vi "SLL DE AI Continuous Engine.vi"(8 "error in (no error)":errorcluster, 11 "Delay (ms)":u32=100) -> (0 "error out":errorcluster)   [LabVIEW 2013]
doc: "Copyright © 2005, Soliton Technologies.\nAll rights reserved."
uses:
  Controls/SLL DE DAQ Engine Options.ctl
  Controls/SLL DE DAQ Engine Channel Types.ctl
  Controls/SLL DE Circular Buffer Options.ctl
  Controls/SLL DE DAQ Global Options.ctl
  Controls/SLL DE DAQ Global Elements.ctl
  Controls/SLL DE DAQ Parameters LV2Global Options.ctl
  <vilib>/DAQmx/configure/timing.llb/DAQmx Timing (Sample Clock).vi
  <vilib>/DAQmx/read.llb/DAQmx Read (Analog 1D Wfm NChan NSamp).vi
  <vilib>/DAQmx/configure/trigger.llb/DAQmx Start Trigger (Digital Edge).vi
panel:
  in  "Data Cluster":T1={"Array of Tasks"=[], "Channel Order"=[], "AI Data"=[], "# Samples"=0, "# Channels"=0, "Time Increments"=[], "AI Cont. Parameters"={"AI Sampling Rate"=1000.0, "MvgAVG Window Size"=1000, "Enable Filter"=TRUE, "Enable MvgAVG"=TRUE}}
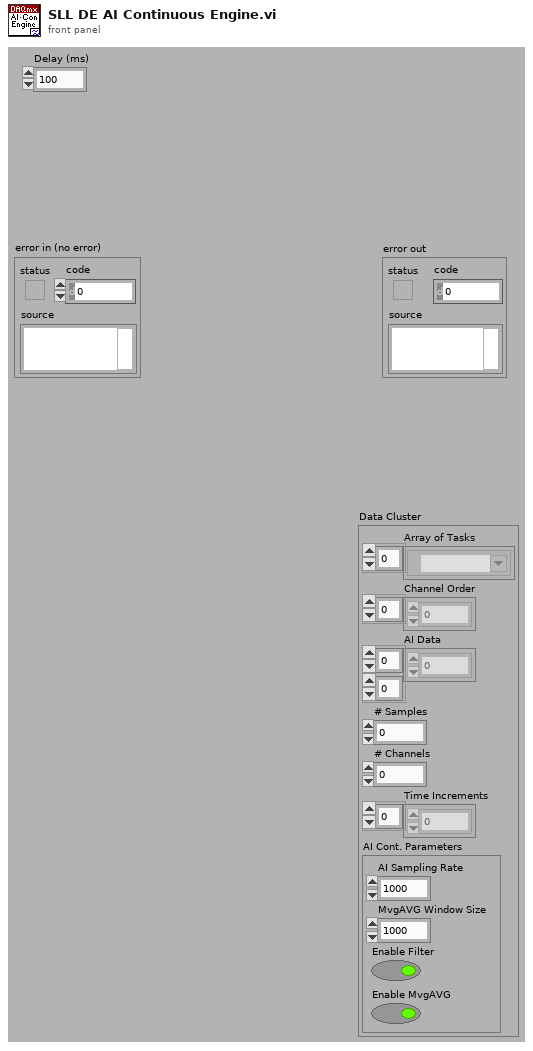
[diagram p1: front panel]
types:
  T1 = cluster{"Array of Tasks":refnum<k21>[], "Channel Order":i32[], "AI Data":dbl[][], "# Samples":i32, "# Channels":i32, "Time Increments":dbl[], "AI Cont. Parameters":cluster{"AI Sampling Rate":dbl, "MvgAVG Window Size":i32, "Enable Filter":bool, "Enable MvgAVG":bool}}
  T2 = typedef "SLL DE DAQ Engine Options.ctl" = enum16{">Init", ">Safe Mode", ">Poll", ">Error", ">Exit", ">Restart", ">DI", ">DO", ">AI", ">AO", ">Start Task", ">Stop Task"}
  T3 = typedef "SLL DE DAQ Parameters LV2Global Options.ctl" = enum16{"Read", "Write"}
  T4 = typedef "SLL DE DAQ Global Options.ctl" = enum16{"Init", "Write 1", "Read 1", "Write Array", "Read Array", "Clear"}
  T5 = typedef "SLL DE Circular Buffer Options.ctl" = enum16{"Initialize", "Init Pointer X", "Write", "Read Single Value", "Read Pointer X (Multi Value)", "Clear Data"}
  T6 = typedef "SLL DE DAQ Engine Channel Types.ctl" = enum16{"Analog Input", "Analog Output", "Digital Input", "Digital Output"}
  T7 = typedef "SLL DE DAQ Global Elements.ctl" = enum16{"AI Error", "AO Error", "DI Error", "DO Error", "AI Restart", "DI Restart", "AI Running", "AO Running", "DI Running", "DO Running", "DAQ Exit?"}
  T8 = typedef "SLL DE DAQ Engine Parameters.ctl" = cluster{"Enable Engines":cluster{"AI Enable":bool, "AO Enable":bool, "DI Enable":bool, "DO Enable":bool}, "DAQ Control Type":cluster{"Analog Input":enum16{"Finite", "Continuous", "Driver"}, "Analog Output":enum16{"Finite", "Continuous", "Driver"}, "Digital Input":enum16{"Finite", "Continuous", "Driver"}, "Digital Output":enum16{"Finite", "Continuous", "Driver"}}, "DAQ Parameters":cluster{"AI Sampling Rate (Samples/Sec)":dbl, "MvgAVG Window Size (# of Points)":i32, "Enable Filter":bool, "Enable MvgAVG":bool, "Circular Buffer Size (Sec)":dbl, "AO Sampling Rate (Samples/Sec)":dbl, "Graph Update Rate (Samples/Sec)":dbl, "File Logging Rate (Samples/Sec)":i32}, "AO Safe Values":cluster{"Analog Outputs Name":T9, "Analog Outputs Safe Value":dbl}[], "DO Safe Values":cluster{"Digital Outputs Name":T10, "Digital Outputs Safe Value":bool}[], "DO Interconnected Lines":cluster{"First DO Line":string, "Second DO Line":string}[], "AI Channels Unit":cluster{"Channel Name":T11, "Channel Type":T12}[], "Units Information":cluster{"Channel Type":T12, "Unit Text":string, "Maximum":dbl, "Minmum":dbl, "Increments":dbl}[]}
  T9 = typedef "SLL DE List of Analog Outputs.ctl" = enum16{"None"}
  T10 = typedef "SLL DE List of Digital Outputs.ctl" = enum16{"STATION1_START TEST", "STATION1_STOP TEST", "STATION1_LIGHT1", "STATION1_LIGHT2", "STATION1_LIGHT3", "STATION1_SELECT_TEST", "STATION2_START TEST", "STATION2_STOP TEST", "STATION2_LIGHT1", "STATION2_LIGHT2", "STATION2_LIGHT3", "STATION2_SELECT_TEST", "STATION3_START TEST", "STATION3_STOP TEST", "STATION3_LIGHT1", "STATION3_LIGHT2", "STATION3_LIGHT3", "STATION3_SELECT_TEST", "STATION4_START TEST", "STATION4_STOP TEST", "STATION4_LIGHT1", "STATION4_LIGHT2", "STATION4_LIGHT3", "STATION4_SELECT_TEST"}
  T11 = typedef "SLL DE List of Analog Inputs.ctl" = enum16{"None"}
  T12 = typedef "SLL DE List of AI Channel Type.ctl" = enum16{"Pressure", "Flow", "Temperature", "Time Scale", "Voltage", "Current", "Frequency", "Sound", "Speed", "Torque", "Distance", "Channel Type 1", "Channel Type 2", "Channel Type 3"}
  T13 = enum16{"Left Button", "Center Button", "Right Button", "Window Close"}
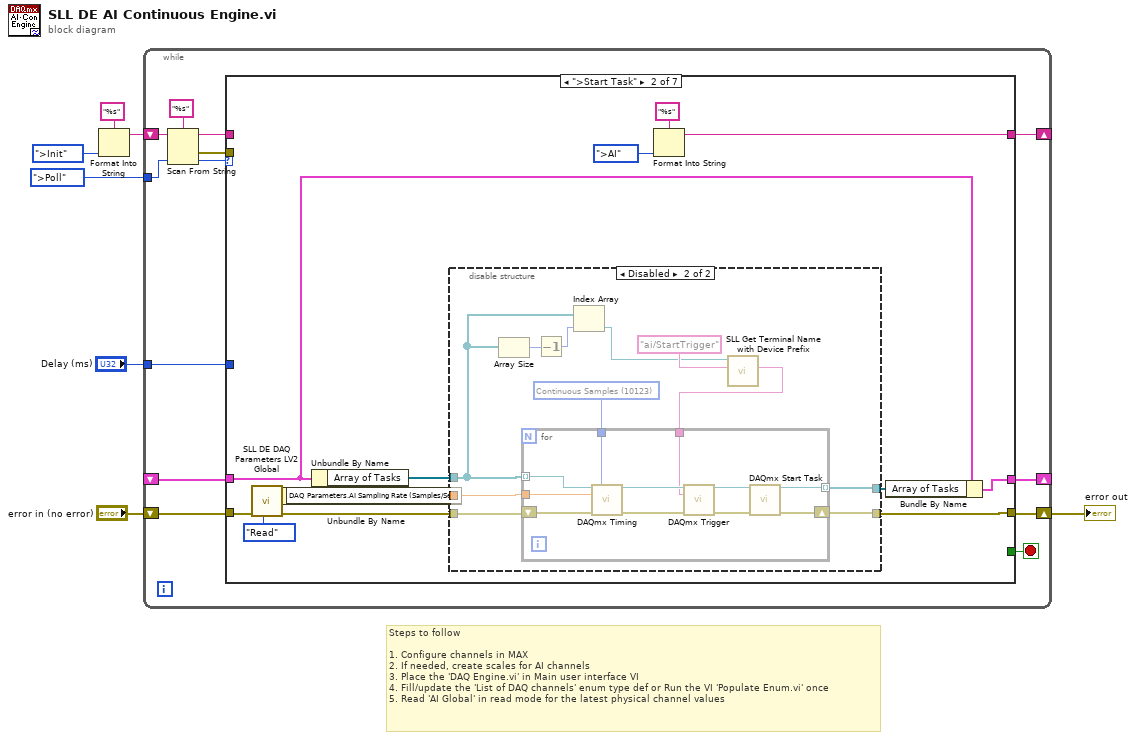
[diagram p0: block diagram]
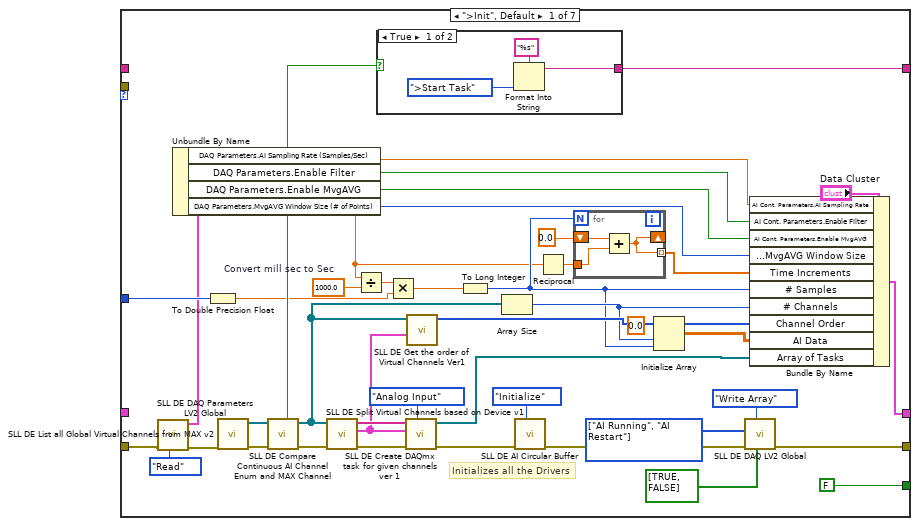
[diagram p2: hidden frame]
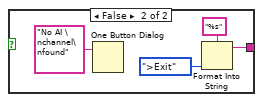
[diagram p3: hidden frame]
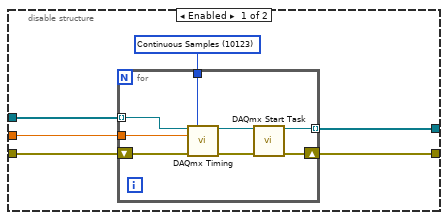
[diagram p4: hidden frame]
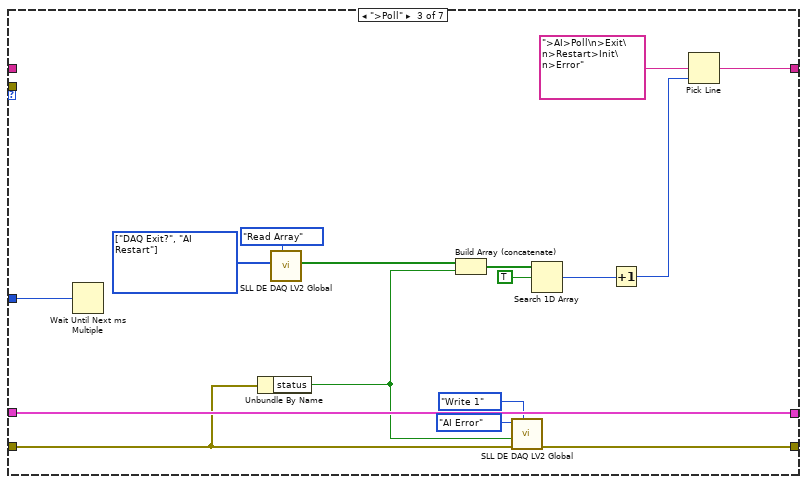
[diagram p5: hidden frame]
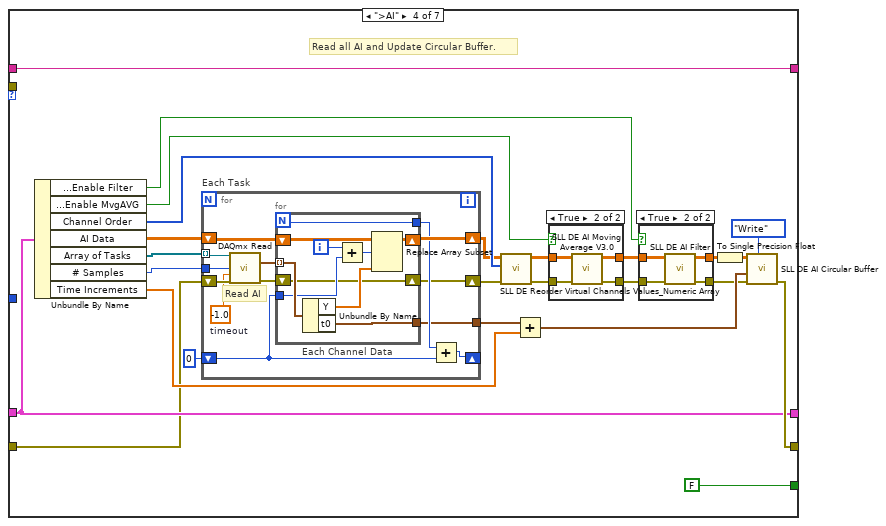
[diagram p6: hidden frame]
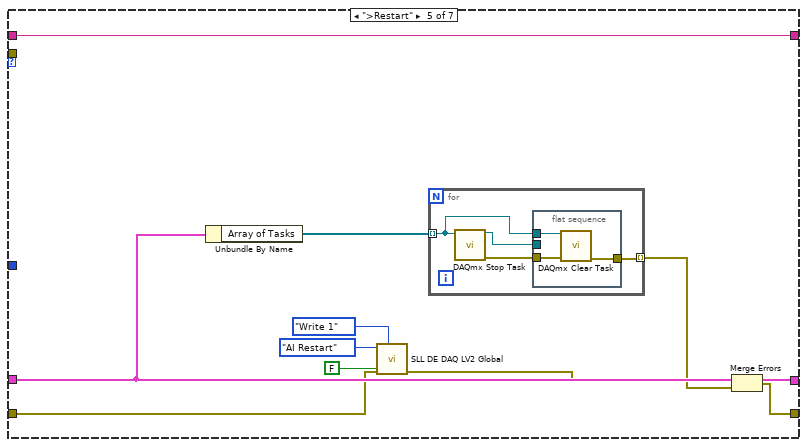
[diagram p9: hidden frame]
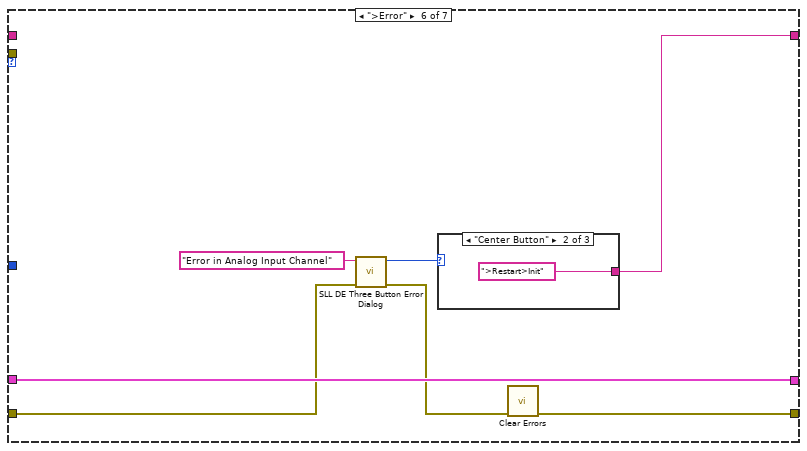
[diagram p10: hidden frame]
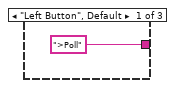
[diagram p11: hidden frame]
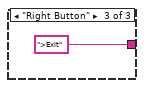
[diagram p12: hidden frame]
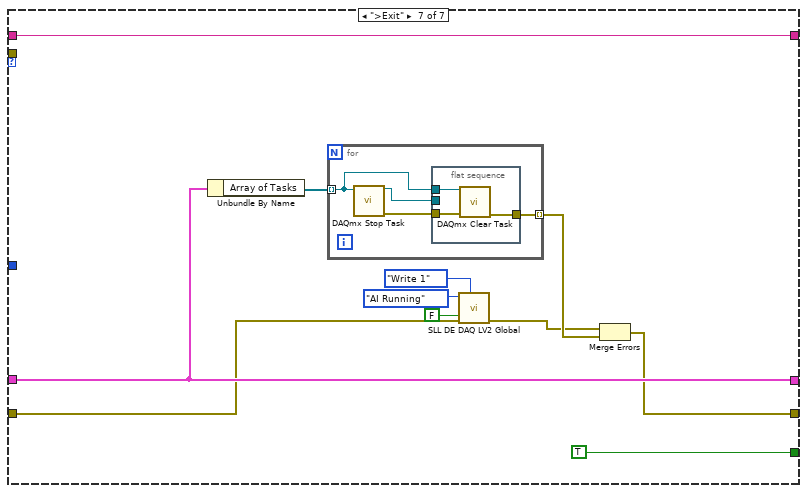
[diagram p13: hidden frame]
diagram:
  # "Steps to follow\n\n1.\tConfigure channels in MAX\n2.\tIf needed, create scales for AI channels\n3.\tPlace the 'DAQ Engine.vi' in Main user interface VI\n4.\tFill/update the 'List of DAQ channels' enum type def or Run the VI 'Populate Enum.vi' once\n5.\tRead 'AI Global' in read mode for the latest physical channel values"
  n1 = Format Into String(format string="%s", SLL_DE_DAQ_Engine_Options.">Init" ("DAQ Options")) -> (resulting string=w3:string)  [unwired: 2 in, 1 out]
  n2 = while {
    shift-right: [w19] -> w6
    shift-left: "error in (no error)" -> [w20]
    shift-right: [w18] -> _
    shift-left: _ -> [w17]
    shift-right: [w13] -> _
    shift-left: w3 -> [w16]
    tunnel: "Delay (ms)" -> [w11]
    tunnel: SLL_DE_DAQ_Engine_Options.">Poll" ("DAQ Options") -> [w9]
    stop <- w12 stop-if-true
    n3 = Scan From String(format string="%s", input string=w16, default 1=w9) -> (remaining string=w15:string, error out=w14:errorcluster, output 1=w10:T2)  [unwired: 2 in, 1 out]
    n4 = case shown="\">Start Task\"" w10 {
      tunnel: w20 -> [w24 w76 w127 w151 w201 w215 w224]
      tunnel: [w56 w81 w126 w159 w197 w217 w229] -> w19
      tunnel: [w62 w82 w137 w156 w206 w220 w232] -> w18
      tunnel: w17 -> [_ w83 w137 w156 w206 w220 w232]
      tunnel: w15 -> [_ _ _ w161 w200 _ w234]
      tunnel: w14 -> [_ _ _ _ _ _ _]
      tunnel: [w59 w78 w131 w161 w200 w216 w234] -> w13
      tunnel: [FALSE _ _ FALSE _ _ TRUE] -> w12
      tunnel: w11 -> [w40 _ w130 _ _ _ _]
      frame ">Init", Default {
        w55 = T7[] [enum."AI Running", enum."AI Restart"] items=["AI Error", "AO Error", "DI Error", "DO Error", "AI Restart", "DI Restart", "AI Running", "AO Running", "DI Running", "DO Running", "DAQ Exit?"] ("Elements Array")
        w42 = 1000.0  # Convert mill sec to Sec
        # "Initializes all the Drivers"
        n5 = call "SLL DE DAQ Parameters LV2 Global.vi"("Option"=SLL_DE_DAQ_Parameters_LV2Global_Options."Read", "Error in (no error)"=w24) -> ("Error out"=w23:errorcluster, "Global Info"=w22:T8)  [unwired: 8 in]
        n6 = Unbundle By Name(w22) -> ("DAQ Parameters.AI Sampling Rate (Samples/Sec)"=w30:dbl, "DAQ Parameters.Enable Filter"=w29:bool, "DAQ Parameters.Enable MvgAVG"=w28:bool, "DAQ Parameters.MvgAVG Window Size (# of Points)"=w27:i32)
        n7 = To Double Precision Float(number=w40) -> (double precision float=w39:dbl)
        n8 = call "SLL DE List all Global Virtual Channels from MAX v2.vi"("error in (no error)"=w23) -> ("error out"=w46:errorcluster, "Analog Input"=w44:refnum<k21>[])  [unwired: 4 in, 5 out]
        n9 = call "SLL DE Compare Continuous AI Channel Enum and MAX Channel.vi"("error in (no error)"=w46, "Analog Input Channels"=w44) -> ("error out"=w45:errorcluster, "Channels Out"=w38:refnum<k21>[], "Pass?"=w43:bool)  [unwired: 7 in]
        n10 = call "SLL DE Split Virtual Channels based on Device v1.vi"("error in (no error)"=w45, "GlobalChans"=w38) -> ("error out"=w51:errorcluster, "Channel Array"=w48:cluster{"Device Channel List":string[]}[], "Devices Names"=w52:string[])  [unwired: 7 in]
        n11 = Divide(x=w30, y=w42) -> (x/y=w41:dbl)
        n12 = case shown="True" w43 {
          tunnel: [w66 w70] -> w59
          frame True {
            n13 = Format Into String(format string="%s", SLL_DE_DAQ_Engine_Options.">Start Task" ("DAQ Options")) -> (resulting string=w66:string)  [unwired: 2 in, 1 out]
          }
          frame False {
            n14 = One Button Dialog(message="No AI \nchannel\nfound") -> ()  [unwired: 1 in, 1 out]
            n15 = Format Into String(format string="%s", SLL_DE_DAQ_Engine_Options.">Exit" ("DAQ Options")) -> (resulting string=w70:string)  [unwired: 2 in, 1 out]
          }
        }
        n16 = Multiply(x=w41, y=w39) -> (x*y=w26:dbl)
        n17 = call "SLL DE Create DAQmx task for given channels ver 1.vi"("Channel Type"=SLL_DE_DAQ_Engine_Channel_Types."Analog Input", "error in (no error)"=w51, "Channel Array"=w48, "Devices Names"=w52) -> ("error out"=w49:errorcluster, "Array of Tasks"=w21:refnum<k21>[])  [unwired: 6 in]
        n18 = call "SLL DE Get the order of Virtual Channels Ver1.vi"("Channel Array"=w48, "Virtial Channels Info"=w38) -> ("Channel Order"=w50:i32[])  [unwired: 8 in, 1 out]
        n19 = To Long Integer(number=w26) -> (32bit integer=w32:i32)
        n20 = Array Size(array=w38) -> (size(s)=w35:i32)
        n21 = call "SLL DE AI Circular Buffer.vi"("Options"=SLL_DE_Circular_Buffer_Options."Initialize" ("AI Option"), "error in (no error)"=w49) -> ("error Out"=w57:errorcluster)  [unwired: 4 in, 5 out]
        n22 = Reciprocal(x=w30) -> (1/x=w33:dbl)
        n23 = for {
          N: w32 -> [_]
          tunnel: w33 -> [w65]
          shift-right: [w63] -> _
          shift-left: 0.0 ("1/x") -> [w64]
          tunnel: [w63] -> w31 mode=indexing
          n24 = Add(x=w64, y=w65) -> (x+y=w63:dbl)
        }
        n25 = Initialize Array(0.0 ("element"), w35, w32) -> (w37:dbl[][])
        n26 = call "SLL DE DAQ LV2 Global.vi"("Status Array In"=bool[] [TRUE, FALSE], "Option"=SLL_DE_DAQ_Global_Options."Write Array", "error in (no error)"=w57, "Elements Array"=w55) -> ("error out"=w56:errorcluster)  [unwired: 5 in, 2 out]
        n27 = Bundle By Name(cluster="Data Cluster", "AI Cont. Parameters.AI Sampling Rate"=w30, "AI Cont. Parameters.Enable Filter"=w29, "AI Cont. Parameters.Enable MvgAVG"=w28, "AI Cont. Parameters.MvgAVG Window Size"=w27, "Time Increments"=w31, "# Samples"=w32, "# Channels"=w35, "Channel Order"=w50, "AI Data"=w37, "Array of Tasks"=w21) -> (w62:T1)
      }
      frame ">Start Task" {
        n28 = call "SLL DE DAQ Parameters LV2 Global.vi"("Option"=SLL_DE_DAQ_Parameters_LV2Global_Options."Read", "Error in (no error)"=w76) -> ("Error out"=w75:errorcluster, "Global Info"=w74:T8)  [unwired: 8 in]
        n29 = Unbundle By Name(w74) -> ("DAQ Parameters.AI Sampling Rate (Samples/Sec)"=w73:dbl)
        n30 = Unbundle By Name(w83) -> ("Array of Tasks"=w85:refnum<k21>[])
        n31 = disable-structure shown="Disabled" {
          disable-tunnel: w85 -> [w90 w106]
          disable-tunnel: [w89 w101] -> w84
          disable-tunnel: w75 -> [w88 w110]
          disable-tunnel: w73 -> [w87 w109]
          disable-tunnel: [w86 w100] -> w81
          frame Enabled {
            w91 = 10123 items=["Finite Samples"=10178, "Continuous Samples"=10123, "Hardware Timed Single Point"=12522] ("sample mode")
            n32 = for {
              tunnel: w91 -> [w96]
              tunnel: w87 -> [w95]
              shift-right: [w97] -> w86
              shift-left: w88 -> [w99]
              tunnel: w90 -> [w93] mode=indexing
              tunnel: [w92] -> w89 mode=indexing
              n33 = call-poly <vilib>:"DAQmx Timing.vi"("task/channels in"=w93, "sample mode"=w96, "rate"=w95, "error in"=w99) -> ("task out"=w94:refnum<k21>, "error out"=w98:errorcluster)  [unwired: 3 in, 7 out]
              n34 = call <vilib>:"DAQmx Start Task.vi"("task/channels in"=w94, "error in"=w98) -> ("task out"=w92:refnum<k21>, "error out"=w97:errorcluster)  [unwired: 12 out]
            }
          }
          frame Disabled {
            w108 = 10123 items=["Finite Samples"=10178, "Continuous Samples"=10123, "Hardware Timed Single Point"=12522] ("sample mode")
            n35 = Array Size(array=w106) -> (size(s)=w105:i32)
            n36 = Decrement(x=w105) -> (x-1=w104:i32)
            n37 = Index Array(array=w106, index=w104) -> (element=w103:refnum<k21>)
            n38 = call "SLL Get Terminal Name with Device Prefix.vi"("Local Terminal Name"="ai/StartTrigger" ("terminal"), "task/channels in"=w103) -> ("Terminal Name with Device Prefix"=w102:tag)  [unwired: 7 in, 2 out]
            n39 = for {
              tunnel: w108 -> [w119]
              tunnel: w109 -> [w118]
              shift-right: [w120] -> w100
              shift-left: w110 -> [w121]
              tunnel: w106 -> [w117] mode=indexing
              tunnel: [w116] -> w101 mode=indexing
              tunnel: w102 -> [w111]
              n40 = call-poly <vilib>:"DAQmx Timing.vi"("task/channels in"=w117, "sample mode"=w119, "rate"=w118, "error in"=w121) -> ("task out"=w114:refnum<k21>, "error out"=w115:errorcluster)  [unwired: 3 in, 7 out]
              n41 = call-poly <vilib>:"DAQmx Trigger.vi"("task/channels in"=w114, "source"=w111, "error in"=w115) -> ("task out"=w112:refnum<k21>, "error out"=w113:errorcluster)  [unwired: 11 in]
              n42 = call <vilib>:"DAQmx Start Task.vi"("task/channels in"=w112, "error in"=w113) -> ("task out"=w116:refnum<k21>, "error out"=w120:errorcluster)  [unwired: 12 out]
            }
          }
        }
        n43 = Format Into String(format string="%s", SLL_DE_DAQ_Engine_Options.">AI" ("DAQ Options")) -> (resulting string=w78:string)  [unwired: 2 in, 1 out]
        n44 = Bundle By Name(cluster=w83, "Array of Tasks"=w84) -> (w82:T1)
      }
      frame ">Poll" {
        w123 = T7[] [enum."DAQ Exit?", enum."AI Restart"] items=["AI Error", "AO Error", "DI Error", "DO Error", "AI Restart", "DI Restart", "AI Running", "AO Running", "DI Running", "DO Running", "DAQ Exit?"] ("Elements Array")
        n45 = Wait Until Next ms Multiple(millisecond multiple=w130) -> ()  [unwired: 1 out]
        n46 = Unbundle By Name(w127) -> ("status"=w125:bool)
        n47 = call "SLL DE DAQ LV2 Global.vi"("Option"=SLL_DE_DAQ_Global_Options."Read Array", "Elements Array"=w123) -> ("Status Array Out"=w122:bool[])  [unwired: 7 in, 2 out]
        n48 = Build Array (concatenate)(w122, w125) -> (w135:bool[])
        n49 = call "SLL DE DAQ LV2 Global.vi"("Option"=SLL_DE_DAQ_Global_Options."Write 1", "error in (no error)"=w127, "Status In"=w125, "Element"=SLL_DE_DAQ_Global_Elements."AI Error") -> ("error out"=w126:errorcluster)  [unwired: 5 in, 2 out]
        n50 = Search 1D Array(1D array=w135, element=TRUE) -> (index of element=w133:i32)  [unwired: 1 in]
        n51 = Increment(x=w133) -> (x+1=w132:i32)
        n52 = Pick Line(multi-line string=">AI>Poll\n>Exit\n>Restart>Init\n>Error", line index=w132) -> (output string=w131:string)  [unwired: 1 in]
      }
      frame ">AI" {
        # "Read all AI and Update Circular Buffer."
        n53 = Unbundle By Name(w156) -> ("AI Cont. Parameters.Enable Filter"=w142:bool, "AI Cont. Parameters.Enable MvgAVG"=w145:bool, "Channel Order"=w157:i32[], "AI Data"=w148:dbl[][], "Array of Tasks"=w149:refnum<k21>[], "# Samples"=w150:i32, "Time Increments"=w154:dbl[])
        n54 = for "Each Task" {
          tunnel: w149 -> [w186] mode=indexing
          shift-right: [w183] -> w141
          shift-left: w148 -> [w184]
          shift-right: [w176] -> w147
          shift-left: w151 -> [w185]
          tunnel: w150 -> [w182]
          shift-right: [w181] -> _
          shift-left: 0 -> [w179]
          tunnel: [w178] -> w146
          w174 = -1.0  # timeout
          # "Read AI"
          n55 = call-poly <vilib>:"DAQmx Read.vi"("task/channels in"=w186, "number of samples per channel"=w182, "timeout"=w174, "error in"=w185) -> ("data"=w175:waveform(dbl)[], "error out"=w177:errorcluster)  [unwired: 9 in, 1 out]
          n56 = for "Each Channel Data" {
            N -> [w191]
            tunnel: w175 -> [w194] mode=indexing
            shift-right: [w195] -> w183
            shift-left: w184 -> [w196]
            tunnel: [w192] -> w178
            tunnel: [w191] -> w180
            tunnel: w179 -> [w190]
            shift-right: [w188] -> w176
            shift-left: w177 -> [w188]
            i -> [w189]
            n57 = Unbundle By Name(w194) -> ("Y"=w193:dbl[], "t0"=w192:timestamp)
            n58 = Add(x=w189, y=w190) -> (x+y=w187:i32)
            n59 = Replace Array Subset(array=w196, new element=w193, index (row)=w187) -> (w195:dbl[][])  [unwired: 1 in]
          }
          n60 = Add(x=w180, y=w179) -> (x+y=w181:i32)
        }
        n61 = call "SLL DE Reorder Virtual Channels Values_Numeric Array.vi"("error in (no error)"=w147, "Channel Order"=w157, "Disordered DI Data"=w141) -> ("error out"=w155:errorcluster, "Ordered DI Data"=w138:dbl[][])  [unwired: 7 in]
        n62 = Add(x=w146, y=w154) -> (x+y=w153:timestamp[])
        n63 = case shown="True" w145 {
          tunnel: w155 -> [w168 w171]
          tunnel: [w168 w170] -> w144
          tunnel: w138 -> [w169 w173]
          tunnel: [w169 w172] -> w143
          frame False {
          }
          frame True {
            n64 = call "SLL DE AI Moving Average V3.0.vi"("error in (no error)"=w171, "Input Array"=w173) -> ("error out"=w170:errorcluster, "Averaged Array"=w172:dbl[][])  [unwired: 8 in]
          }
        }
        n65 = case shown="True" w142 {
          tunnel: w144 -> [w162 w165]
          tunnel: [w162 w164] -> _
          tunnel: w143 -> [w163 w167]
          tunnel: [w163 w166] -> w140
          frame False {
          }
          frame True {
            n66 = call "SLL DE AI Filter.vi"("error in (no error)"=w165, "Raw Data"=w167) -> ("error out"=w164:errorcluster, "Filtered Avg Data"=w166:dbl[][])  [unwired: 8 in]
          }
        }
        n67 = To Single Precision Float(number=w140) -> (single precision float=w139:sgl[][])
        n68 = call "SLL DE AI Circular Buffer.vi"("Options"=SLL_DE_Circular_Buffer_Options."Write" ("AI Option"), "error in (no error)"=w144, "Time In"=w153, "Input Data"=w139) -> ("error Out"=w159:errorcluster)  [unwired: 2 in, 5 out]
      }
      frame ">Restart" {
        n69 = Unbundle By Name(w206) -> ("Array of Tasks"=w205:refnum<k21>[])
        n70 = call "SLL DE DAQ LV2 Global.vi"("Option"=SLL_DE_DAQ_Global_Options."Write 1", "error in (no error)"=w201, "Status In"=FALSE, "Element"=SLL_DE_DAQ_Global_Elements."AI Restart") -> ("error out"=w199:errorcluster)  [unwired: 5 in, 2 out]
        n71 = for {
          tunnel: w205 -> [w210] mode=indexing
          tunnel: [w207] -> w198 mode=indexing
          n72 = call <vilib>:"DAQmx Stop Task.vi"("task/channels in"=w210) -> ("task out"=w209:refnum<k21>, "error out"=w208:errorcluster)  [unwired: 13 in]
          n73 = flat-sequence {
            tunnel: w210 -> [w213]
            tunnel: w209 -> [_]
            tunnel: w208 -> [w212]
            tunnel: [w211] -> w207
            frame #0 {
              n74 = call <vilib>:"DAQmx Clear Task.vi"("task in"=w213, "error in"=w212) -> ("error out"=w211:errorcluster)  [unwired: 13 in]
            }
          }
        }
        n75 = Merge Errors(w199, w198) -> (w197:errorcluster)
      }
      frame ">Error" {
        n76 = call "SLL DE Three Button Error Dialog.vi"("Error In"=w215, "Window Title"="Error in Analog Input Channel") -> ("Error Out"=w214:errorcluster, "Which Button?"=w218:T13)  [unwired: 8 in]
        n77 = case shown="\"Center Button\"" w218 {
          tunnel: [">Poll" ("Window Title") ">Restart>Init" ("Window Title") ">Exit" ("Window Title")] -> w216
          frame "Left Button", Default {
          }
          frame "Center Button" {
          }
          frame "Right Button" {
          }
        }
        n78 = call <vilib>:"Clear Errors.vi"("error in (no error)"=w214) -> ("error out"=w217:errorcluster)  [unwired: 6 in]
      }
      frame ">Exit" {
        n79 = Unbundle By Name(w232) -> ("Array of Tasks"=w231:refnum<k21>[])
        n80 = for {
          tunnel: w231 -> [w238] mode=indexing
          tunnel: [w235] -> w230 mode=indexing
          n81 = call <vilib>:"DAQmx Stop Task.vi"("task/channels in"=w238) -> ("task out"=w237:refnum<k21>, "error out"=w236:errorcluster)  [unwired: 13 in]
          n82 = flat-sequence {
            tunnel: w238 -> [w241]
            tunnel: w237 -> [_]
            tunnel: w236 -> [w239]
            tunnel: [w240] -> w235
            frame #0 {
              n83 = call <vilib>:"DAQmx Clear Task.vi"("task in"=w241, "error in"=w239) -> ("error out"=w240:errorcluster)  [unwired: 13 in]
            }
          }
        }
        n84 = call "SLL DE DAQ LV2 Global.vi"("Option"=SLL_DE_DAQ_Global_Options."Write 1", "error in (no error)"=w224, "Status In"=FALSE, "Element"=SLL_DE_DAQ_Global_Elements."AI Running") -> ("error out"=w227:errorcluster)  [unwired: 5 in, 2 out]
        n85 = Merge Errors(w227, w230) -> (w229:errorcluster)
      }
    }
  }
  "error out" <- w6
